vi "Reset.vi"(8 "error in (no error)":errorcluster, 11 "ProdType_1 in":refnum<class "ProdType_1.lvclass">) -> (0 "error out":errorcluster, 1 "Status":string, 3 "ProdType_1 out":refnum<class "ProdType_1.lvclass">)   [LabVIEW 2020, in "I2COUSB.lvlib" / "ProdType_1.lvclass"]
doc: "Reset I2C BUS"
uses:
  ProdType_1.lvclass
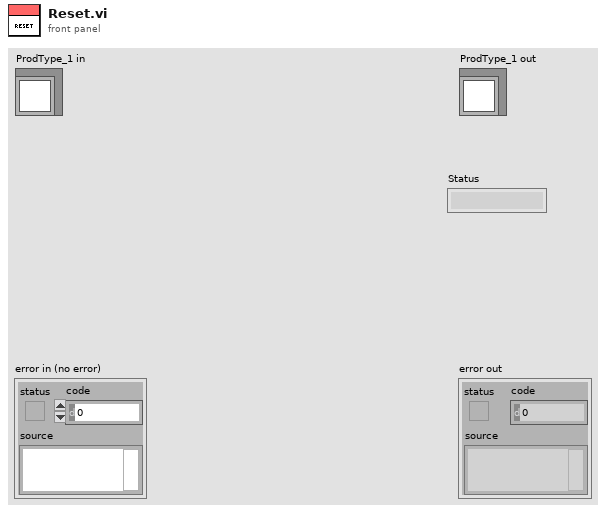
[diagram p1: front panel]
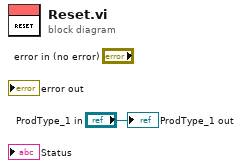
[diagram p0: block diagram]
diagram:
  "ProdType_1 out" <- "ProdType_1 in"
